vi "Modder.vi"() -> ()   [LabVIEW 2013]
uses:
  Tools/mod_tag.ctl
  Tools/Line.ctl
  <vilib>/gmath/NI_Gmath.lvlib
panel:
  in  "Line":T1
  out "error out":errorcluster
  out "String Formats":string[](array[string])
  in  "Send Button":bool
  in  "Save Button":bool
  in  "Save":path
  in  "Stop Button":bool
  in  "Make Button":bool
  in  "Tab Control":enum32{"Sequence", "Mod TAGs"}(tab)
  in  "Template SEQ":T1
  out "Output SEQs":T1[](array[typedef])
  out "Built":i32
  out "Progress":u8(slide)=100 max=15 scale=0.0..100.0 scale format="%.2f"
  in  "defualt format":string="%0.4g"
  in  "Reorder":bool
  out "Mod Vars":string[](array[string])
  out "Permutations":dbl[][](array[numeric]) format="%#_8g"
  in  "Build Arrays":T2[](array[typedef]) {"Steps" min=1 step=1}
  out "size(s)":i32[](array[numeric])
  # "Modder"
  # "Use $math ($) to start (end) expressions,\ne.g. $math (XX +1 ) / XY $"
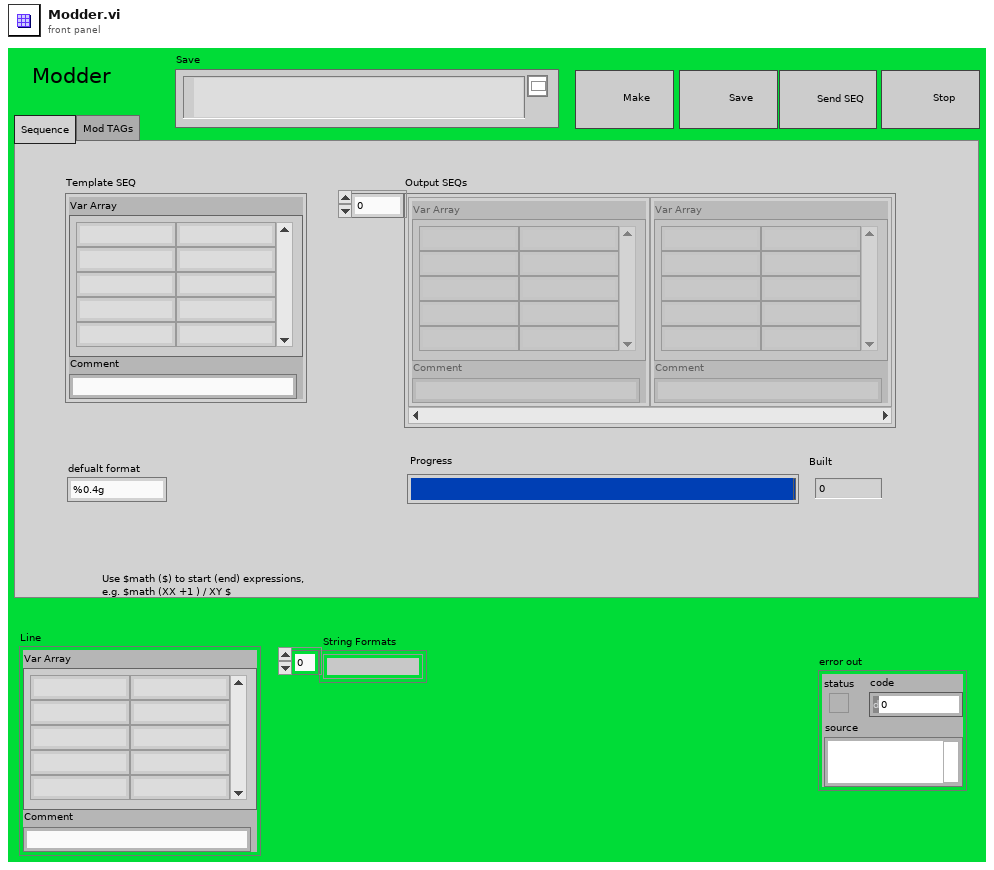
[diagram p1: front panel]
types:
  T1 = typedef "Line.ctl" = cluster{"Var Array":string[][], "Comment":string}
  T2 = typedef "mod_tag.ctl" = cluster{"TAG":string, "Array":dbl[], "f(x)":string, "Steps":i32, "Build":bool, "Reorder Each":bool, "Format":string}
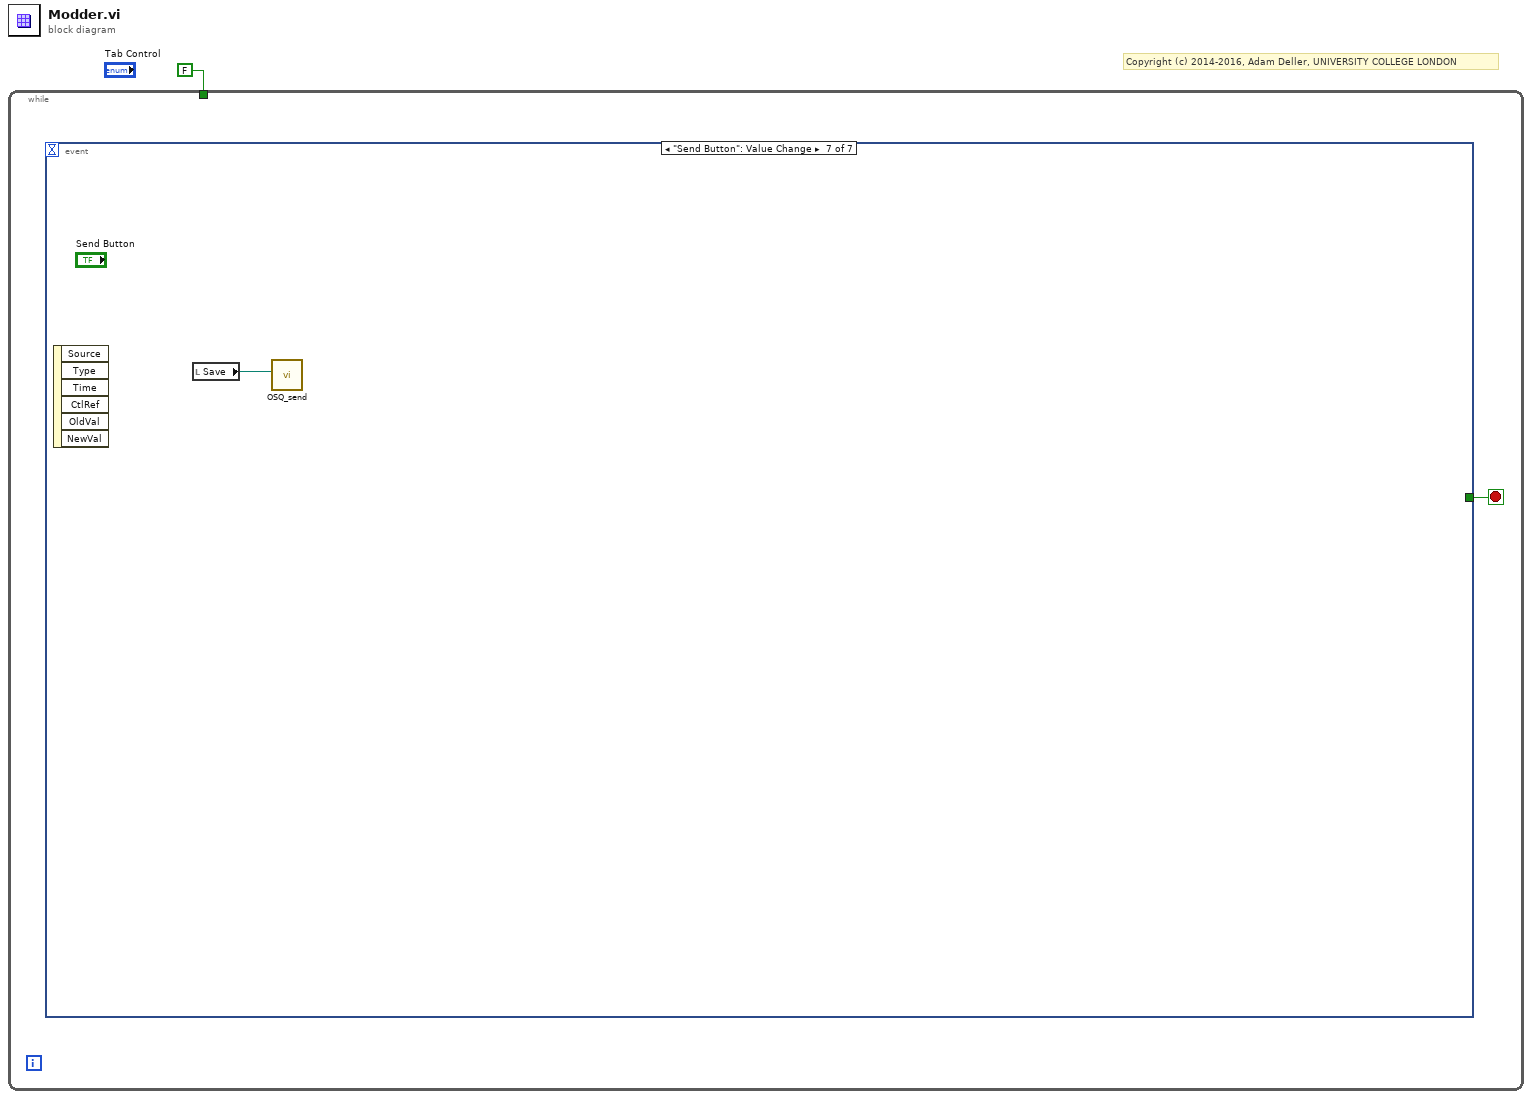
[diagram p0: block diagram]
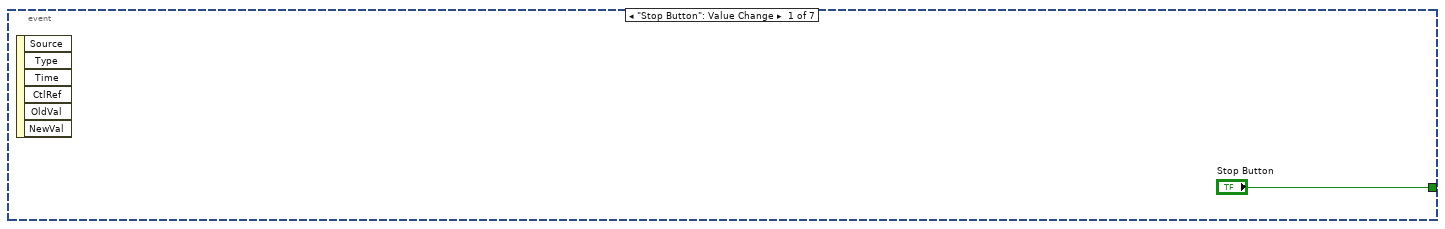
[diagram p2: hidden frame]
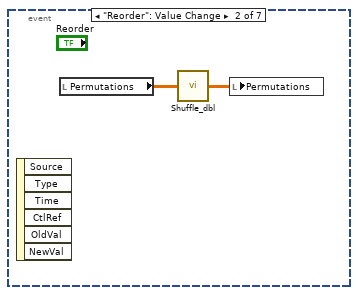
[diagram p3: hidden frame]
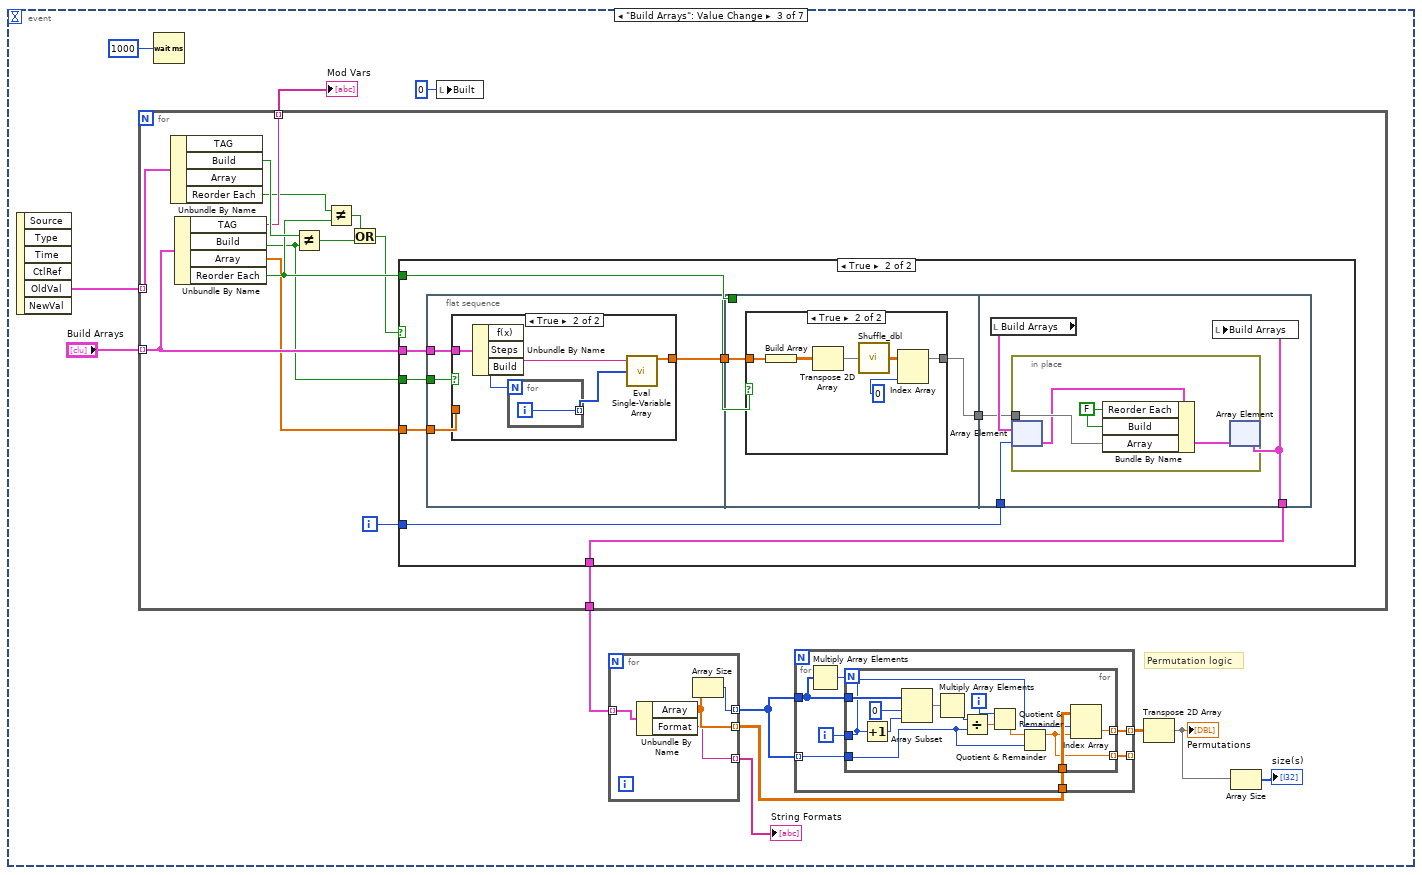
[diagram p4: hidden frame]
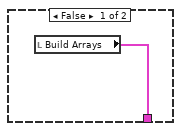
[diagram p5: hidden frame]
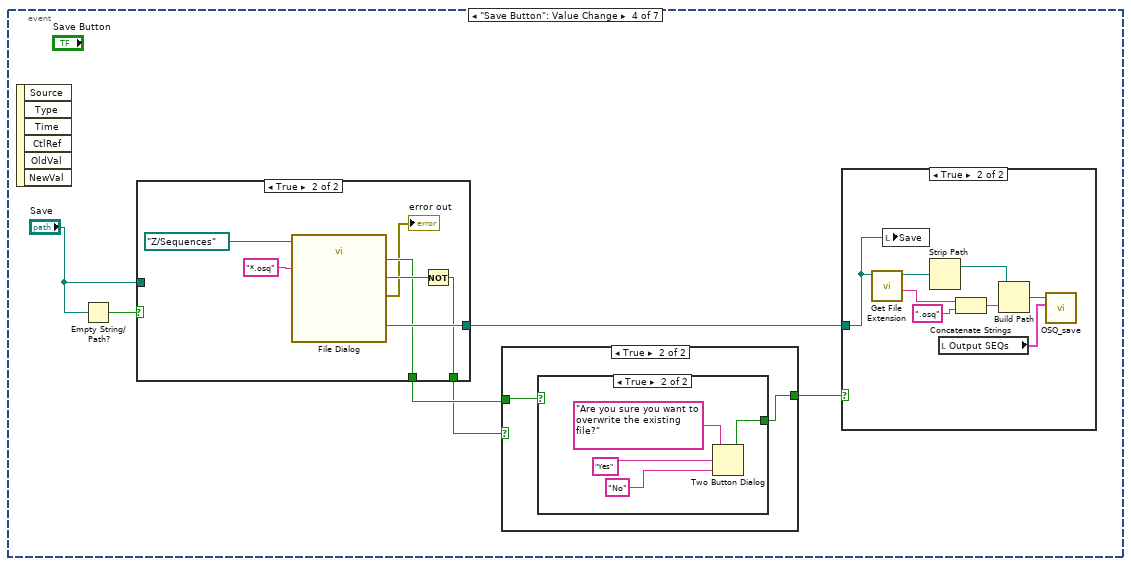
[diagram p8: hidden frame]
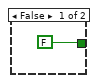
[diagram p9: hidden frame]
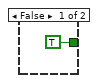
[diagram p10: hidden frame]
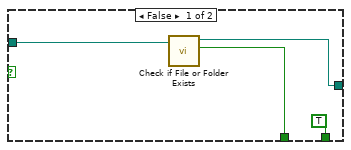
[diagram p11: hidden frame]
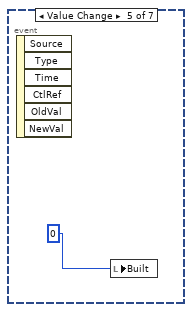
[diagram p13: hidden frame]
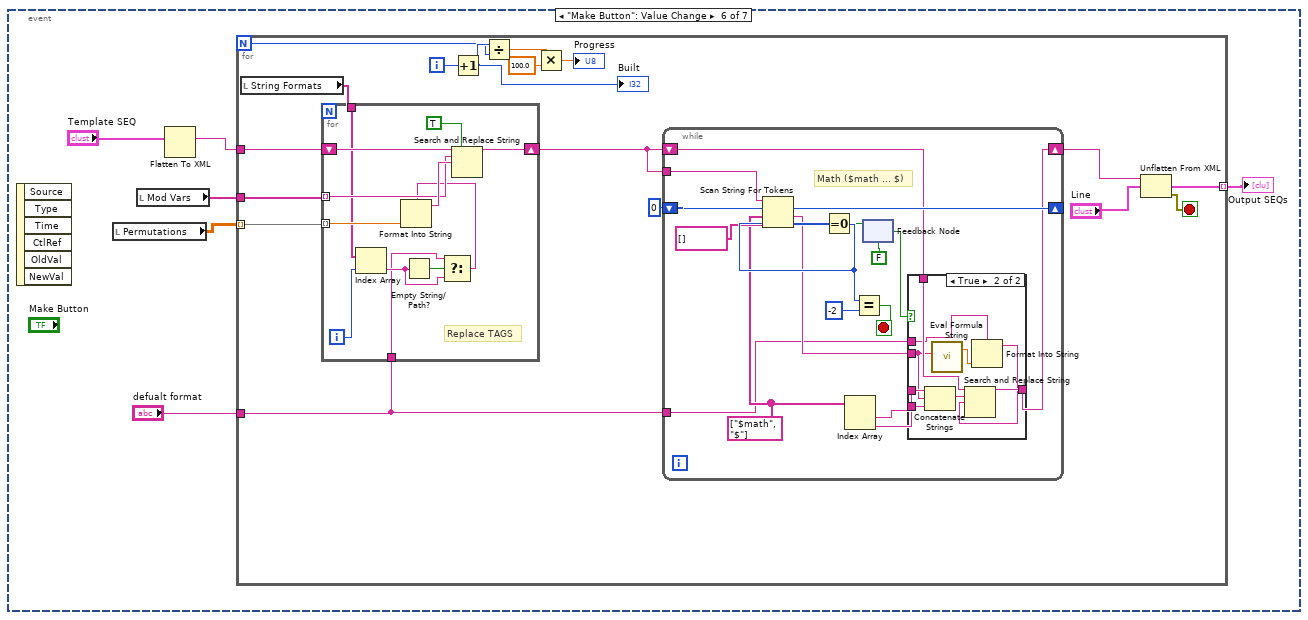
[diagram p14: hidden frame]
diagram:
  # "Copyright (c) 2014-2016, Adam Deller, UNIVERSITY COLLEGE LONDON"
  n1 = while {
    tunnel: FALSE ("Done") -> [_]
    stop <- w2 stop-if-true
    n2 = event shown="[6] \"Send Button\": Value Change" {
      selector: _ -> [_ _ _ _ _ _ _]
      dyn-events: _ -> [_ _ _ _ _ _ _]
      timeout: _ -> [_ _ _ _ _ _ _]
      tunnel: ["Stop Button" _ _ _ _ _ _] -> w2
      event "Stop Button": Value Change {
        n3 = event-data() -> ()  [unwired: 1 in, 6 out]
      }
      event "Reorder": Value Change {
        n4 = event-data() -> ()  [unwired: 1 in, 6 out]
        n5 = local read "Permutations"() -> (w5:dbl[][])
        n6 = call "Shuffle_dbl.vi"("Array IN"=w5) -> ("Array OUT"=w4:dbl[][])
        n7 = local write "Permutations"(w4) -> ()
      }
      event "Build Arrays": Value Change {
        # "Permutation logic"
        n8 = event-data() -> ("OldVal"=w17:T2[])  [unwired: 1 in, 5 out]
        n9 = for {
          tunnel: "Build Arrays" -> [w53] mode=indexing
          tunnel: w17 -> [w54] mode=indexing
          tunnel: [w50] -> w15 mode=indexing
          tunnel: [w42] -> w9
          i -> [w52]
          n10 = Unbundle By Name(w54) -> ("Build"=w51:bool, "Reorder Each"=w49:bool)  [unwired: 2 out]
          n11 = Unbundle By Name(w53) -> ("TAG"=w50:string, "Build"=w43:bool, "Array"=w45:dbl[], "Reorder Each"=w48:bool)
          n12 = Not Equal?(x=w51, y=w43) -> (x != y?=w46:bool)
          n13 = Not Equal?(x=w49, y=w48) -> (x != y?=w47:bool)
          n14 = Or(x=w47, y=w46) -> (x .or. y?=w44:bool)
          n15 = case shown="True" w44 {
            tunnel: w53 -> [_ w63]
            tunnel: w52 -> [_ w62]
            tunnel: w45 -> [_ w57]
            tunnel: w48 -> [_ w60]
            tunnel: [w55 w58] -> w42
            tunnel: w43 -> [_ w56]
            frame False {
              n16 = local read "Build Arrays"() -> (w55:T2[])
            }
            frame True {
              n17 = flat-sequence {
                tunnel: w63 -> [w67]
                tunnel: [w66] -> w61
                tunnel: w57 -> [w65]
                tunnel: w56 -> [w64]
                tunnel: w61 -> [w76]
                tunnel: w60 -> [w77]
                tunnel: [w75] -> w59
                tunnel: w62 -> [w88]
                tunnel: [w85] -> w58
                tunnel: w59 -> [w86]
                frame #0 {
                  n18 = case shown="True" w64 {
                    tunnel: w67 -> [_ w73]
                    tunnel: [w68 w69] -> w66
                    tunnel: w65 -> [w68 _]
                    frame False {
                    }
                    frame True {
                      n19 = Unbundle By Name(w73) -> ("f(x)"=w72:string, "Steps"=w71:i32)  [unwired: 1 out]
                      n20 = for {
                        N: w71 -> [_]
                        tunnel: [w74] -> w70 mode=indexing
                        i -> [w74]
                      }
                      n21 = call <vilib>:"Eval Single-Variable Array.vi"("X Values"=w70, "formula"=w72) -> ("Y Values"=w69:dbl[])  [unwired: 1 in, 1 out]
                    }
                  }
                }
                frame #1 {
                  n22 = case shown="True" w77 {
                    tunnel: w76 -> [w78 w84]
                    tunnel: [w78 w82] -> w75
                    frame False {
                    }
                    frame True {
                      n23 = Build Array(w84) -> (w81:dbl[][])
                      n24 = Transpose 2D Array(2D array=w81) -> (transposed array=w80:dbl[][])
                      n25 = call "Shuffle_dbl.vi"("Array IN"=w80) -> ("Array OUT"=w83:dbl[][])
                      n26 = Index Array(array=w83, index (col)=0 ("disabled index (col)")) -> (element=w82:dbl[])  [unwired: 1 in]
                    }
                  }
                }
                frame #2 {
                  n27 = local read "Build Arrays"() -> (w87:T2[])
                  n28 = in-place {
                    in-place-border: w86 -> [w92]
                    w89 = FALSE ("Use")
                    n29 = in-place-array #1(w87, w88) -> (w91:T2)
                    n30 = Bundle By Name(cluster=w91, "Reorder Each"=w89, "Build"=w89, "Array"=w92) -> (w90:T2)
                    n31 = in-place-array #1(w90) -> (w85:T2[])  [unwired: 1 out]
                  }
                  n32 = local write "Build Arrays"(w85) -> ()
                }
              }
            }
          }
        }
        "Mod Vars" <- w15
        n33 = Wait (ms)(milliseconds to wait=1000) -> ()  [unwired: 1 out]
        n34 = local write "Built"(0 ("Built")) -> ()
        n35 = for {
          tunnel: [w20] -> w10 mode=indexing
          tunnel: [w21] -> w11 mode=indexing
          tunnel: w9 -> [w19] mode=indexing
          tunnel: [w18] -> w6 mode=indexing
          n36 = Unbundle By Name(w19) -> ("Array"=w21:dbl[], "Format"=w18:string)
          n37 = Array Size(array=w21) -> (size(s)=w20:i32)
        }
        "String Formats" <- w6
        n38 = for {
          tunnel: w10 -> [w27]
          tunnel: w10 -> [w25] mode=indexing
          tunnel: w11 -> [w24]
          tunnel: [w23] -> w12 mode=indexing
          tunnel: [w22] -> _ mode=indexing
          i -> [w28]
          n39 = Multiply Array Elements(1:w27) -> (0:w26:i32)
          n40 = for {
            N: w26 -> [_]
            tunnel: w27 -> [w40]
            tunnel: w28 -> [w30]
            tunnel: w25 -> [w35]
            tunnel: w24 -> [w33]
            tunnel: [w32] -> w23 mode=indexing
            tunnel: [w29] -> w22 mode=indexing
            i -> [w31]
            n41 = Increment(x=w30) -> (x+1=w38:i32)
            n42 = Array Subset(array=w40, index=0, length=w38) -> (w39:i32[])
            n43 = Multiply Array Elements(1:w39) -> (0:w37:i32)
            n44 = Divide(x=w37, y=w35) -> (x/y=w36:dbl)
            n45 = Quotient & Remainder(x=w31, y=w36) -> (floor(x/y)=w34:dbl)  [unwired: 1 out]
            n46 = Quotient & Remainder(x=w34, y=w35) -> (x-y*floor(x/y)=w29:dbl)  [unwired: 1 out]
            n47 = Index Array(array=w33, index (row)=w30, index (col)=w29) -> (element=w32:dbl)
          }
        }
        n48 = Transpose 2D Array(2D array=w12) -> (transposed array=w8:dbl[][])
        "Permutations" <- w8
        n49 = Array Size(array=w8) -> (size(s)=→"size(s)":i32[])
      }
      event "Save Button": Value Change {
        n50 = event-data() -> ()  [unwired: 1 in, 6 out]
        n51 = Empty String/Path?(string/path="Save") -> (empty?=w98:bool)
        n52 = case shown="True" w98 {
          tunnel: "Save" -> [w110 _]
          tunnel: [w108 w115] -> w93
          tunnel: [w109 w112] -> w97
          tunnel: [TRUE w113] -> w96
          frame False {
            n53 = call <vilib>:"Check if File or Folder Exists.vi"("path"=w110) -> ("file or folder exists?"=w109:bool, "dup path"=w108:path)  [unwired: 8 in, 1 out]
          }
          frame True {
            n54 = call "File Dialog"("start path"=path "Z:/Sequences", "pattern (all files)"="*.osq") -> ("selected path"=w115:path, "exists"=w112:bool, "cancelled"=w114:bool, "error out"=→"error out":errorcluster)  [unwired: 10 in]
            n55 = Not(x=w114) -> (.not. x?=w113:bool)
          }
        }
        n56 = case shown="True" w96 {
          tunnel: w97 -> [_ w101]
          tunnel: [FALSE w100] -> w95
          frame False {
          }
          frame True {
            n57 = case shown="True" w101 {
              tunnel: [TRUE ("T button?") w104] -> w100
              frame False {
              }
              frame True {
                n58 = Two Button Dialog(message="Are you sure you want to overwrite the existing file?", 1:"No" ("Right Button Text (\"Cancel\")"), 2:"Yes" ("T button name (\"OK\")")) -> (T button?=w104:bool)
              }
            }
          }
        }
        n59 = case shown="True" w95 {
          tunnel: w93 -> [_ w118]
          frame False {
          }
          frame True {
            n60 = call <vilib>:"Get File Extension.vi"("file"=w118) -> ("filename without extension"=w122:string, "dup file"=w120:path)  [unwired: 7 in, 2 out]
            n61 = local write "Save"(w118) -> ()
            n62 = Strip Path(path=w120) -> (stripped path=w119:path)  [unwired: 1 out]
            n63 = local read "Output SEQs"() -> (w125:T1[])
            n64 = Concatenate Strings(w122, ".osq" ("string")) -> (w123:string)
            n65 = Build Path(base path=w119, name or relative path=w123) -> (appended path=w121:path)
            n66 = call "OSQ_save.vi"("SEQs"=w125, "Save"=w121) -> ()  [unwired: 8 in, 2 out]
          }
        }
      }
      event Value Change {
        n67 = event-data() -> ()  [unwired: 1 in, 6 out]
        n68 = local write "Built"(u8 0 ("Slide")) -> ()
      }
      event "Make Button": Value Change {
        n69 = event-data() -> ()  [unwired: 1 in, 6 out]
        n70 = local read "Permutations"() -> (w132:dbl[][])
        n71 = local read "Mod Vars"() -> (w131:string[])
        n72 = Flatten To XML(anything="Template SEQ") -> (xml string=w129:string)
        n73 = for {
          N -> [w144]
          tunnel: w129 -> [w147]
          tunnel: w131 -> [w149]
          tunnel: w132 -> [w148] mode=indexing
          tunnel: [w139] -> w128 mode=indexing
          tunnel: "defualt format" -> [w133]
          i -> [w146]
          stop <- w138 stop-if-true
          n74 = local read "String Formats"() -> (w134:string[])
          n75 = for {
            tunnel: w149 -> [w183] mode=indexing
            tunnel: w148 -> [w188] mode=indexing
            shift-right: [w186] -> w136
            shift-left: w147 -> [w185]
            tunnel: w134 -> [w182]
            tunnel: w133 -> [w177]
            i -> [w181]
            # "Replace TAGS"
            n76 = Index Array(array=w182, index=w181) -> (element=w179:string)
            n77 = Empty String/Path?(string/path=w179) -> (empty?=w180:bool)
            n78 = Select(t=w177, s=w180, f=w179) -> (s? t:f=w178:string)
            n79 = Format Into String(format string=w178, w188) -> (resulting string=w184:string)  [unwired: 2 in, 1 out]
            n80 = Search and Replace String(replace all?=TRUE ("replace all? (F)"), input string=w185, search string=w183, replace string=w184) -> (result string=w186:string)  [unwired: 4 in, 3 out]
          }
          n81 = Increment(x=w146) -> (x+1=w145:i32)
          "Built" <- w145
          n82 = Divide(x=w145, y=w144) -> (x/y=w143:dbl)
          n83 = Multiply(x=w143, y=100.0) -> (x*y=→"Progress":dbl)
          n84 = while {
            shift-right: [w165] -> _
            shift-left: 0 ("offset past token") -> [w164]
            tunnel: w136 -> [w166]
            shift-right: [w151] -> w135
            shift-left: w136 -> [w152]
            tunnel: w133 -> [w150]
            stop <- w162 stop-if-true
            w156 = string[] ["$math", "$"] ("delimiters (\\s,\\t,\\r,\\n) 2")
            # "Math ($math ... $)"
            n85 = Scan String For Tokens(6:string[] [] ("delimiters (\\s,\\t,\\r,\\n)"), 7:w156, 8:w164, 9:w166) -> (0:w161:i32, 1:w153:string, 2:w165:i32)  [unwired: 2 in, 1 out]
            n86 = Equal To 0?(x=w161) -> (x = 0?=w160:bool)
            n87 = Index Array(array=w156) -> (element #1=w155:string, element #2=w154:string)  [unwired: 2 in]
            n88 = Equal?(x=w161, y=-2) -> (x = y?=w162:bool)
            n89 = feedback-in #2(w160) -> ()
            n90 = feedback #2(FALSE) -> (w157:bool)
            n91 = case shown="True" w157 {
              tunnel: w153 -> [_ w171]
              tunnel: w155 -> [_ w176]
              tunnel: w154 -> [_ w175]
              tunnel: w152 -> [w167 w173]
              tunnel: [w167 w172] -> w151
              tunnel: w150 -> [_ w168]
              frame False {
              }
              frame True {
                n92 = Concatenate Strings(w176, w171, w175) -> (w174:string)
                n93 = call <vilib>:"Eval Formula String.vi"("formula"=w171) -> ("y value"=w169:dbl)  [unwired: 1 in, 1 out]
                n94 = Format Into String(format string=w168, w169) -> (resulting string=w170:string)  [unwired: 2 in, 1 out]
                n95 = Search and Replace String(input string=w173, search string=w174, replace string=w170) -> (result string=w172:string)  [unwired: 5 in, 3 out]
              }
            }
          }
          n96 = Unflatten From XML(xml string=w135, type="Line") -> (value=w139:T1, error out=w138:errorcluster)  [unwired: 1 in]
        }
        "Output SEQs" <- w128
      }
      event "Send Button": Value Change {
        n97 = event-data() -> ()  [unwired: 1 in, 6 out]
        n98 = local read "Save"() -> (w189:path)
        n99 = call "OSQ_send.vi"("Sequence File"=w189) -> ()  [unwired: 11 in]
      }
    }
  }
